vi "oil valves.vi"() -> ()   [LabVIEW 2017]
panel:
  in  "Boolean":bool
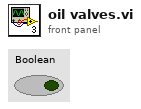
[diagram p1: front panel]
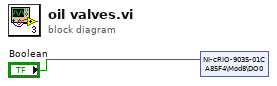
[diagram p0: block diagram]
diagram:
  n1 = shared-variable "NI-cRIO-9035-01CA85F4\\Mod8\\DO0"("Boolean") -> ()  [unwired: 1 in, 1 out]
